vi "prepBreakIn_toplvl.vi"(5 "which manipulator":T1(ring), 7 "Slide Refnum":refnum<vi>, 8 "error in (no error)":errorcluster, 10 "Break In Pressure (mbar)":dbl=-350.0, 11 "Pressure box control in":T2={"Pressure box COM"="COM7", "pressure box type"=enum."ProportionAir", "High pos pressure (mBar)"=0.0, "Low pos pressure (mBar)"=0.0, "Vacuum pressure (mBar)"=0.0, "calibration"=enum."mightenRig"}) -> (0 "error out":errorcluster, 3 "Pressure box control out":T2)   [LabVIEW 2015]
uses:
  controls/arduino_pressure_setting.ctl
  controls/proportionAir_cmds.ctl
  controls/pressure_box_type.ctl
  controls/pressure_box_control.ctl
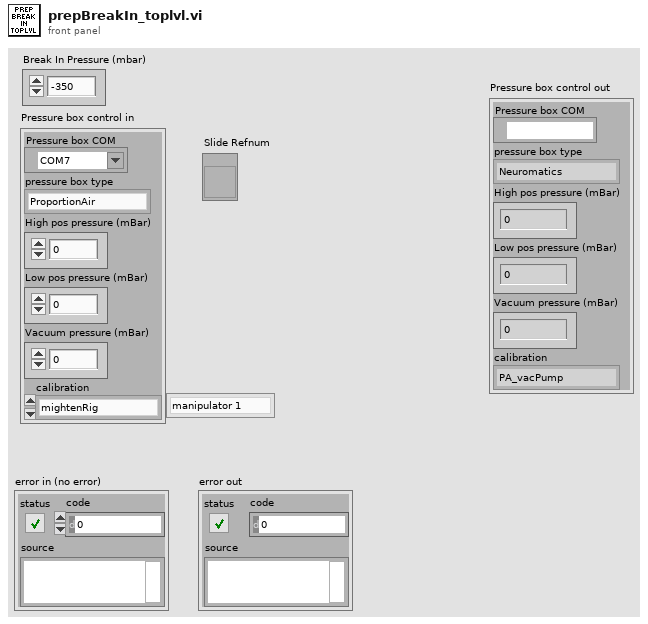
[diagram p1: front panel]
types:
  T1 = enum16{"manipulator 1", "manipulator 2", "manipulator 3", "manipulator 4"}
  T2 = typedef "pressure_box_control.ctl" = cluster{"Pressure box COM":refnum<visa-resource-name>, "pressure box type":T3, "High pos pressure (mBar)":dbl, "Low pos pressure (mBar)":dbl, "Vacuum pressure (mBar)":dbl, "calibration":enum16{"PA_vacPump", "PA_venturi", "Neuromatics", "ilyaRig", "mightenRig"}}
  T3 = typedef "pressure_box_type.ctl" = enum16{"Neuromatics", "ProportionAir", "Demo box", "N-ProportionAir"}
  T4 = typedef "arduino_pressure_setting.ctl" = enum16{"High Positive Pressure", "Low Positive Pressure", "Atmospheric Pressure", "Low Vacuum", "High Vacuum", "Break In", "Puff"}
  T5 = typedef "proportionAir_cmds.ctl" = enum16{"Set P", "Switch to Atm", "Switch to Regulator", "Pulse", "WC"}
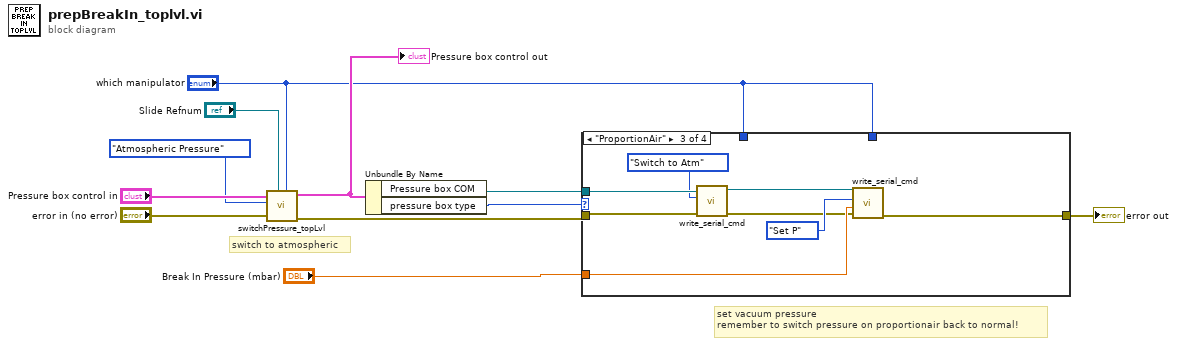
[diagram p0: block diagram]
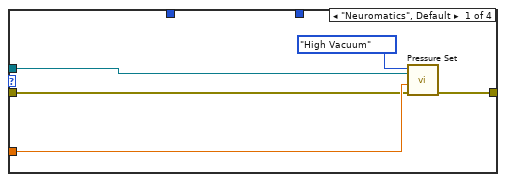
[diagram p2: hidden frame]
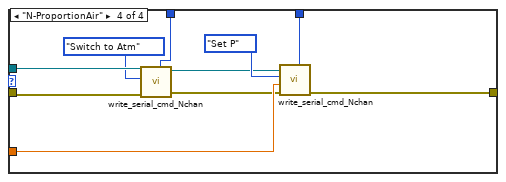
[diagram p4: hidden frame]
diagram:
  # "set vacuum pressure\nremember to switch pressure on proportionair back to normal!"
  # "switch to atmospheric"
  n1 = call "switchPressure_topLvl.vi"("which manipulator"="which manipulator", "Slide Refnum"="Slide Refnum", "error in"="error in (no error)", "pressure setting"=arduino_pressure_setting."Atmospheric Pressure", "Pressure box control in"="Pressure box control in") -> ("error out"=w2:errorcluster, "Pressure box control out"=w4:T2)  [unwired: 5 in]
  "Pressure box control out" <- w4
  n2 = Unbundle By Name(w4) -> ("Pressure box COM"=w10:refnum<visa-resource-name>, "pressure box type"=w11:T3)
  n3 = case shown="\"ProportionAir\"" w11 {
    tunnel: w2 -> [w12 w17 w21 w31]
    tunnel: [w16 w17 w23 w33] -> w9
    tunnel: w10 -> [w14 _ w22 w30]
    tunnel: "Break In Pressure (mbar)" -> [w13 _ w24 w34]
    tunnel: "which manipulator" -> [_ _ _ w32]
    tunnel: "which manipulator" -> [_ _ _ w26]
    frame "Neuromatics", Default {
      n4 = call "Pressure Set.vi"("error in"=w12, "Val"=w13, "Pressure Box COM"=w14, "arduino pressure setting"=arduino_pressure_setting."High Vacuum") -> ("error out"=w16:errorcluster)  [unwired: 6 in, 1 out]
    }
    frame "Demo box" {
    }
    frame "ProportionAir" {
      n5 = call "write_serial_cmd.vi"("error in"=w21, "pressure command"=proportionAir_cmds."Switch to Atm", "Pressure Box COM"=w22) -> ("error out"=w20:errorcluster, "Pressure Box COM out"=w18:refnum<visa-resource-name>)  [unwired: 7 in]
      n6 = call "write_serial_cmd.vi"("error in"=w20, "pressure set (mBar)"=w24, "pressure command"=proportionAir_cmds."Set P", "Pressure Box COM"=w18) -> ("error out"=w23:errorcluster)  [unwired: 6 in, 1 out]
    }
    frame "N-ProportionAir" {
      n7 = call "write_serial_cmd_Nchan.vi"("which manipulator"=w26, "error in"=w31, "pressure command"=proportionAir_cmds."Switch to Atm", "Pressure Box COM"=w30) -> ("error out"=w28:errorcluster, "Pressure Box COM out"=w29:refnum<visa-resource-name>)  [unwired: 6 in]
      n8 = call "write_serial_cmd_Nchan.vi"("which manipulator"=w32, "error in"=w28, "arg 1"=w34, "pressure command"=proportionAir_cmds."Set P", "Pressure Box COM"=w29) -> ("error out"=w33:errorcluster)  [unwired: 5 in, 1 out]
    }
  }
  "error out" <- w9
